vi "Initialize1.vi"(8 "error in (no error)":errorcluster, 11 "device data model in":refnum<class "Standard Data Model1.lvclass">) -> (0 "error out":errorcluster, 3 "device data model out":refnum<class "Standard Data Model1.lvclass">)   [LabVIEW 2021, in "NI_modbus_upd.lvlib" / "Standard Data Model1.lvclass"]
doc: "This VI initializes the device data model."
uses:
  Standard Data Model1.lvclass
  Standard Data Model1.lvclass/Standard Data Model1.ctl
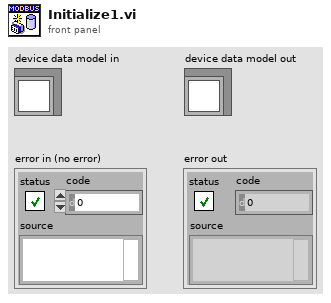
[diagram p1: front panel]
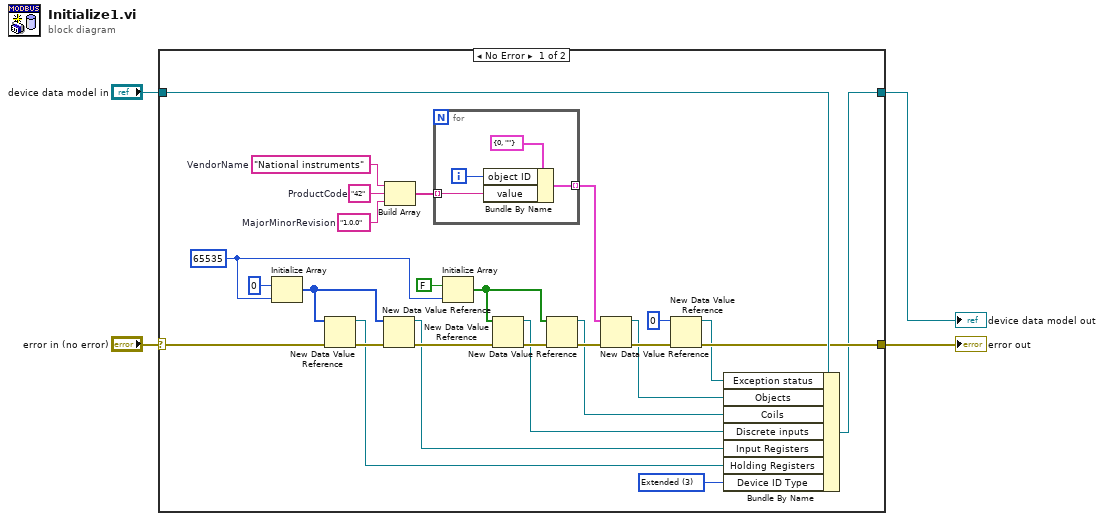
[diagram p0: block diagram]
diagram:
  n1 = case shown="No Error" "error in (no error)" {
    selector: "error in (no error)" -> [w5 w36]
    tunnel: "device data model in" -> [w25 w37]
    tunnel: [w14 w36] -> w2
    tunnel: [w13 w37] -> w1
    frame No Error {
      w7 = u8 3 items=["Basic"=1, "Regular "=2, "Extended"=3] ("Read Device ID Code")
      w26 = "1.0.0"  # MajorMinorRevision
      w28 = "42"  # ProductCode
      w27 = "National instruments"  # VendorName
      w29 = u16 65535
      n2 = Initialize Array(u16 0 ("Numeric"), w29) -> (w19:u16[])
      n3 = New Data Value Reference(data value=w19, error in=w5) -> (data value reference=w12:refnum<data-value>, error out=w21:errorcluster)
      n4 = New Data Value Reference(data value=w19, error in=w21) -> (data value reference=w11:refnum<data-value>, error out=w22:errorcluster)
      n5 = Build Array(w27, w28, w26) -> (w24:string[])
      n6 = for {
        tunnel: w24 -> [w33] mode=indexing
        tunnel: [w32] -> w18 mode=indexing
        i -> [w34]
        n7 = Bundle By Name(cluster=cluster{"object ID":u8, "value":string} {"object ID"=0, "value"=""} ("Cluster"), "object ID"=w34, "value"=w33) -> (w32:cluster{"object ID":u8, "value":string})
      }
      n8 = Initialize Array(FALSE ("Boolean"), w29) -> (w20:bool[])
      n9 = New Data Value Reference(data value=w20, error in=w22) -> (data value reference=w10:refnum<data-value>, error out=w23:errorcluster)
      n10 = New Data Value Reference(data value=w20, error in=w23) -> (data value reference=w9:refnum<data-value>, error out=w17:errorcluster)
      n11 = New Data Value Reference(data value=w18, error in=w17) -> (data value reference=w8:refnum<data-value>, error out=w16:errorcluster)
      n12 = New Data Value Reference(data value=u8 0, error in=w16) -> (data value reference=w6:refnum<data-value>, error out=w14:errorcluster)
      n13 = Bundle By Name(cluster=w25, "Exception status"=w6, "Objects"=w8, "Coils"=w9, "Discrete inputs"=w10, "Input Registers"=w11, "Holding Registers"=w12, "Device ID Type"=w7) -> (w13:refnum<class "Standard Data Model1.lvclass">)
    }
    frame Error {
    }
  }
  "error out" <- w2
  "device data model out" <- w1
